vi "StartandConnectCore.vi"(8 "error in (no error)":errorcluster, 10 "Service Details":T1, 11 "MicronGRPCClient in":refnum<class "MicronGRPCClient.lvclass">) -> (0 "error out":errorcluster, 3 "MicronGRPCClient out":refnum<class "MicronGRPCClient.lvclass">)   [LabVIEW 2019, in "MicronGRPCClient.lvclass"]
uses:
  MicronGRPCClient.lvclass
  Base/Client/Typedefs/ServiceDetails.ctl
  MicronCLI/Typedefs/ServiceDetails.ctl
  a738a202-2849-4230-803a-5db153b72c03.vi
  MicronCLI/MicronCLI.lvclass
  Base/Client/MicronClient.lvclass
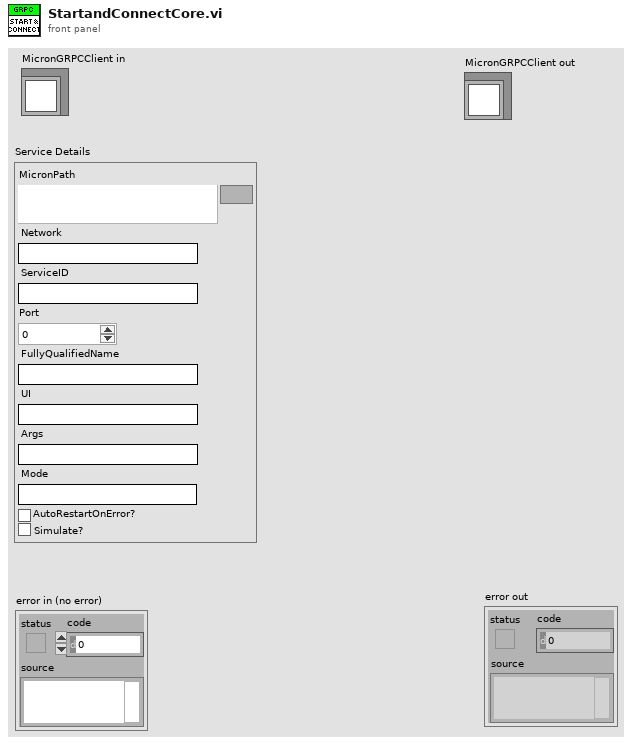
[diagram p1: front panel]
types:
  T1 = typedef "MicronClient.lvclass/ServiceDetails.ctl" = cluster{"MicronPath":path, "Network":string, "ServiceID":string, "Port":i32, "FullyQualifiedName":string, "UI":string, "Args":string, "Mode":string, "AutoRestartOnError?":bool, "Simulate?":bool}
  T2 = typedef "MicronCLI.lvclass/ServiceDetails.ctl" = cluster{"Network":string, "ServiceID":string}
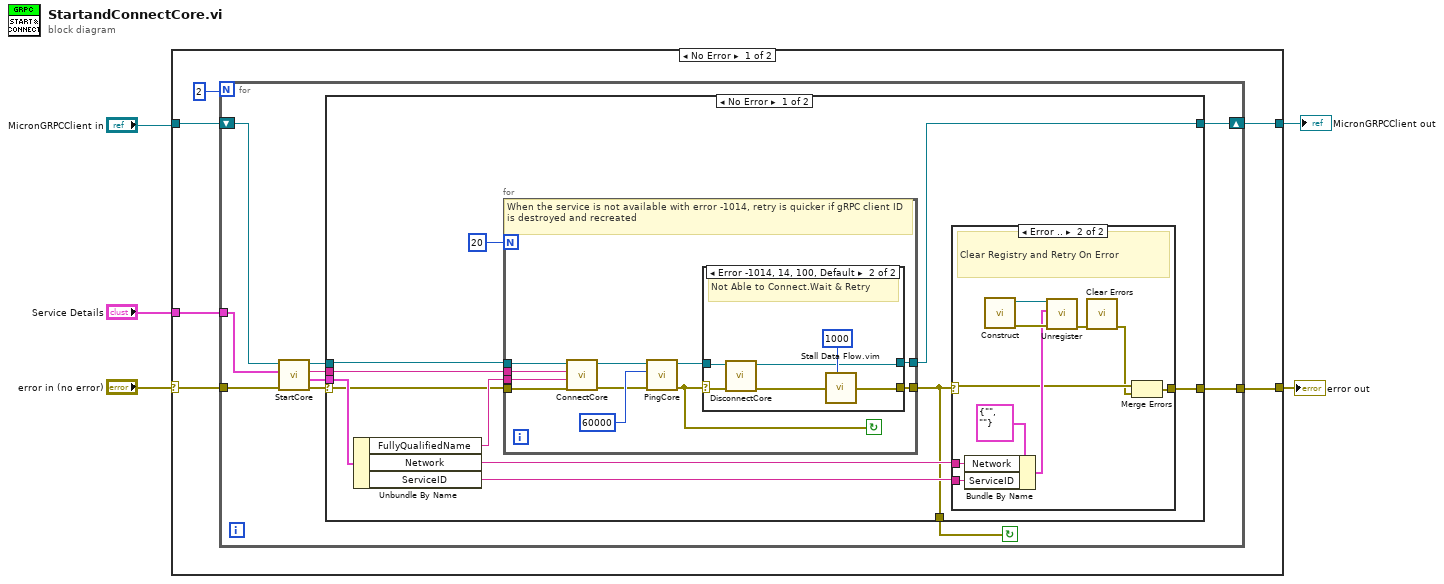
[diagram p0: block diagram]
diagram:
  n1 = case shown="No Error" "error in (no error)" {
    selector: "error in (no error)" -> [w10 w66]
    tunnel: [w7 w66] -> w5
    tunnel: [w9 w65] -> w4
    tunnel: "MicronGRPCClient in" -> [w11 w65]
    tunnel: "Service Details" -> [w8 _]
    frame No Error {
      n2 = for {
        N: 2 -> [_]
        tunnel: w10 -> [w20]
        tunnel: w8 -> [w18]
        shift-right: [w19] -> w9
        shift-left: w11 -> [w21]
        tunnel: [w13] -> w7
        stop <- w12 continue-if-true
        n3 = call-dynamic "StartCore.vi"("error in (no error)"=w20, "Service Details In"=w18, "MicronGRPCClient in"=w21) -> ("error out"=w17:errorcluster, "Service Details Out"=w15:T1, "Connection String"=w14:string, "MicronGRPCClient out"=w16:refnum<class "MicronGRPCClient.lvclass">)  [unwired: 5 in]
        n4 = case shown="No Error" w17 {
          selector: w17 -> [w23 w63]
          tunnel: [w22 w64] -> w19
          tunnel: w16 -> [w24 w64]
          tunnel: w15 -> [w31 _]
          tunnel: w14 -> [w25 _]
          tunnel: [w28 w63] -> w13
          tunnel: [w27 _] -> w12
          frame No Error {
            n5 = Unbundle By Name(w31) -> ("FullyQualifiedName"=w26:string, "Network"=w30:string, "ServiceID"=w29:string)
            n6 = for {
              N: 20 -> [_]
              tunnel: [w53] -> w27
              tunnel: w26 -> [w51]
              tunnel: w25 -> [w50]
              tunnel: w24 -> [w49]
              tunnel: w23 -> [w48]
              tunnel: [w44] -> w22
              stop <- w54 continue-if-true
              # "When the service is not available with error -1014, retry is quicker if gRPC client ID is destroyed and recreated"
              n7 = call-dynamic "ConnectCore.vi"("error in (no error)"=w48, "Fully Qualified Name"=w51, "Connection String"=w50, "GRPCClient in"=w49) -> ("error out"=w46:errorcluster, "GRPCClient out"=w47:refnum<class "MicronGRPCClient.lvclass">)  [unwired: 6 in]
              n8 = call-dynamic "PingCore.vi"("error in (no error)"=w46, "Timeout (ms)"=60000, "MicronGRPCClient in"=w47) -> ("error out"=w54:errorcluster, "MicronGRPCClient out"=w45:refnum<class "MicronGRPCClient.lvclass">)  [unwired: 6 in, 1 out]
              n9 = case shown="Error -1014, 14, 100, Default" w54 {
                selector: w54 -> [w56 w60]
                tunnel: [w56 w62] -> w53
                tunnel: w45 -> [w55 w59]
                tunnel: [w55 w57] -> w44
                frame No Error {
                }
                frame Error, Default {
                  # "Not Able to Connect.Wait & Retry"
                  n10 = call-dynamic "DisconnectCore.vi"("error in (no error)"=w60, "GRPCClient in"=w59) -> ("error out"=w58:errorcluster, "GRPCClient out"=w57:refnum<class "MicronGRPCClient.lvclass">)  [unwired: 8 in]
                  n11 = call "Stall Data Flow.vim"("value in"=w58, "milliseconds to wait"=u32 1000) -> ("value out"=w62:errorcluster)  [unwired: 1 out]
                }
              }
            }
            n12 = case shown="Error .." w27 {
              selector: w27 -> [w33 w36]
              tunnel: [w33 w37] -> w28
              tunnel: w30 -> [_ w40]
              tunnel: w29 -> [_ w39]
              frame No Error {
              }
              frame Error {
                # "Clear Registry and Retry On Error"
                n13 = Bundle By Name(cluster=T2 {"Network"="", "ServiceID"=""} ("Service"), "Network"=w40, "ServiceID"=w39) -> (w38:T2)
                n14 = call "Construct.vi"() -> ("error out"=w43:errorcluster, "MicronCLI out"=w42:refnum<class "MicronCLI.lvclass">)  [unwired: 9 in, 1 out]
                n15 = call-dynamic "Unregister.vi"("error in (no error)"=w43, "Service"=w38, "MicronCLI in"=w42) -> ("error out"=w35:errorcluster)  [unwired: 7 in, 1 out]
                n16 = call <vilib>:"Clear Errors.vi"("error in (no error)"=w35) -> ("error out"=w34:errorcluster)  [unwired: 5 in, 1 out]
                n17 = Merge Errors(w36, w34) -> (w37:errorcluster)
              }
            }
          }
          frame Error {
          }
        }
      }
    }
    frame Error {
    }
  }
  "error out" <- w5
  "MicronGRPCClient out" <- w4
